vi "Clean.vi"(0 "Component in":refnum<class "Component.lvclass">) -> (4 "Component out":refnum<class "Component.lvclass">)   [LabVIEW 2017, in "CL_G3_VIComponentBuilder.lvlib" / "Component.lvclass"]
doc: "Invokes the \"clean\" routine for all exports in this Component."
uses:
  Component.lvclass
  Component.lvclass/Component.ctl
  Accessors/Read Component Operations Errors.vi
  Exports/Exports/Export.lvclass
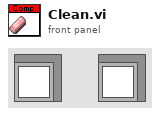
[diagram p1: front panel]
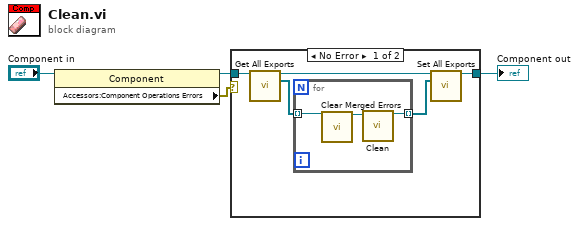
[diagram p0: block diagram]
diagram:
  n1 = property class="Component"(reference="Component in") -> (reference out=w2:refnum<class "Component.lvclass">, "Accessors:Component Operations Errors"=w1:errorcluster)  [unwired: 1 in, 1 out]
  n2 = case shown="No Error" w1 {
    tunnel: [w9 w13] -> w4
    tunnel: w2 -> [w5 w13]
    frame No Error {
      n3 = call "Get All Exports.vi"("Component in"=w5) -> ("Component out"=w7:refnum<class "Component.lvclass">, "Exports"=w8:refnum<class "Export.lvclass">[])  [unwired: 13 in]
      n4 = for {
        tunnel: w8 -> [w11] mode=indexing
        tunnel: [w12] -> w6 mode=indexing
        n5 = call "Clear Merged Errors.vi"("Export in"=w11) -> ("Export out"=w10:refnum<class "Export.lvclass">)  [unwired: 12 in, 2 out]
        n6 = call-dynamic "Clean.vi"("Export in"=w10) -> ("Export out"=w12:refnum<class "Export.lvclass">)  [unwired: 14 in]
      }
      n7 = call "Set All Exports.vi"("Component in"=w7, "Exports"=w6) -> ("Component out"=w9:refnum<class "Component.lvclass">)  [unwired: 13 in]
    }
    frame Error {
    }
  }
  "Component out" <- w4
